vi "New.vi"   [LabVIEW 2026]
panel:
  # "Brand new VI"
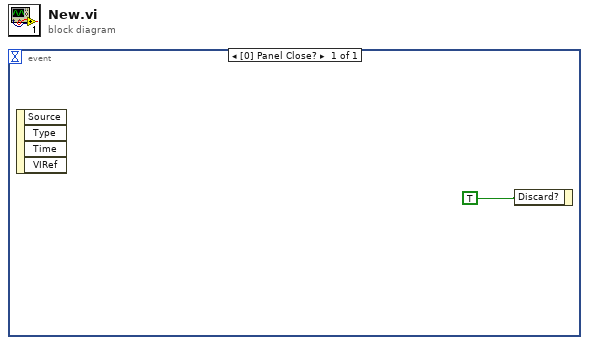
[diagram p0: block diagram]
diagram:
  n1 = event shown="[0] Panel Close?" {
    selector: _ -> [_]
    dyn-events: _ -> [_]
    timeout: _ -> [_]
    event Panel Close? {
      n2 = event-data() -> ()  [unwired: 1 in, 4 out]
      n3 = event-data("Discard?"=TRUE) -> ()  [unwired: 1 in, 1 out]
    }
  }
